vi "SUPERMARKET PROJECT SAVE DATA TO EXCEL.vi"() -> ()   [LabVIEW 2021]
uses:
  <vilib>/Utility/file.llb/Write Delimited Spreadsheet (string).vi
panel:
  in  "?":enum32{"Page 1", "Page 2"}(tab)
  in  "OK Button":bool
  in  "Username":string
  in  "Password":string
  in  "file path (dialog if empty) 2":path
  in  "stop":bool
  in  "Number 01":dbl
  in  "Number 02":dbl
  out "Answer":dbl
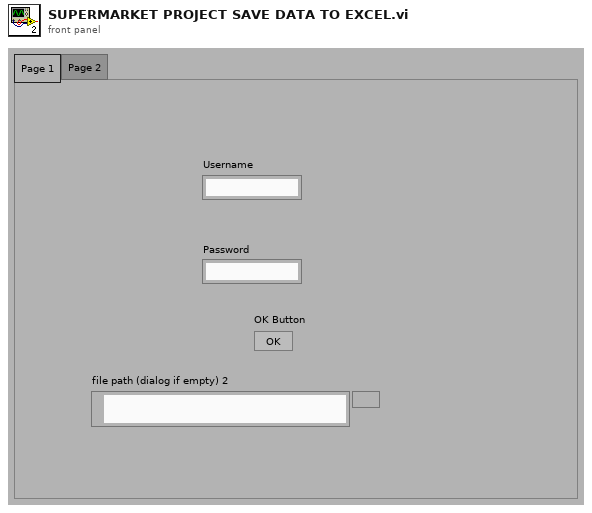
[diagram p1: front panel]
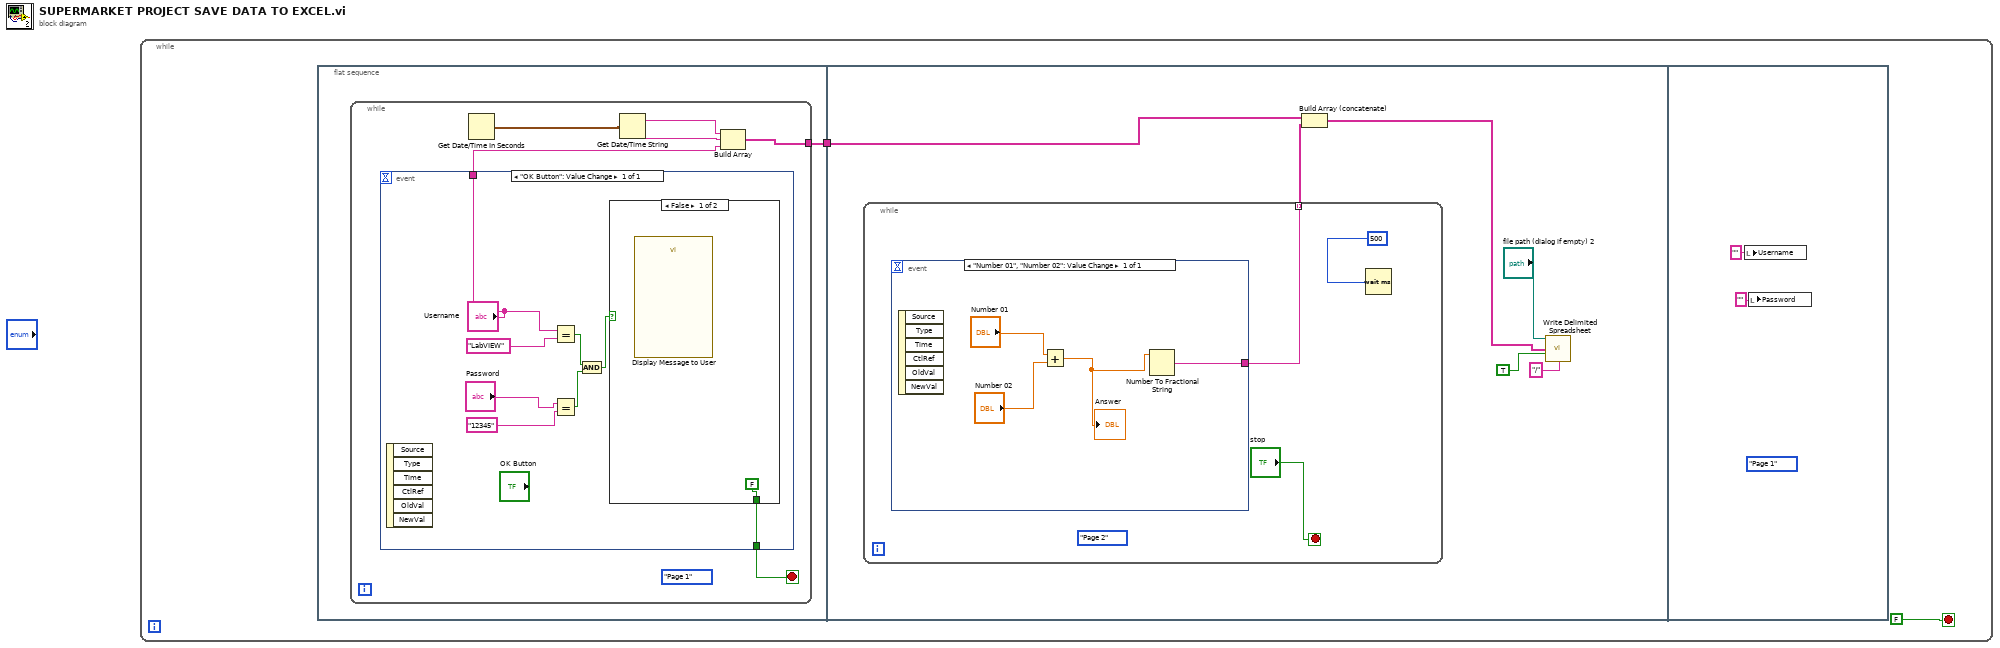
[diagram p0: block diagram]
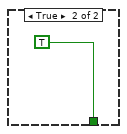
[diagram p2: hidden frame]
diagram:
  n1 = while {
    stop <- FALSE stop-if-true
    n2 = flat-sequence {
      tunnel: [w3] -> w1
      tunnel: w1 -> [w25]
      frame #0 {
        n3 = while {
          tunnel: [w7] -> w3
          stop <- w5 stop-if-true
          (unwired) enum32{"Page 1", "Page 2"}."Page 1"
          n4 = event shown="[0] \"OK Button\": Value Change" {
            selector: _ -> [_]
            dyn-events: _ -> [_]
            timeout: _ -> [_]
            tunnel: ["Username"] -> w4
            tunnel: [w10] -> w5
            event "OK Button": Value Change {
              n5 = event-data() -> ()  [unwired: 1 in, 6 out]
              n6 = Equal?(x="Username", y="LabVIEW") -> (x = y?=w14:bool)
              n7 = Equal?(x="Password", y="12345") -> (x = y?=w13:bool)
              n8 = And(x=w14, y=w13) -> (x .and. y?=w15:bool)
              n9 = case shown="False" w15 {
                tunnel: [FALSE TRUE] -> w10
                frame False {
                  n10 = call "Display Message to User"() -> ()  [unwired: 10 in, 2 out]
                }
                frame True {
                }
              }
            }
          }
          n11 = Get Date/Time In Seconds() -> (seconds since 1Jan1904=w9:timestamp)
          n12 = Get Date/Time String(seconds (now)=w9) -> (date string=w8:string, time string=w6:string)  [unwired: 2 in]
          n13 = Build Array(w8, w6, w4) -> (w7:string[])
        }
      }
      frame #1 {
        n14 = while {
          tunnel: [w27] -> w24 mode=indexing
          stop <- "stop" stop-if-true
          (unwired) enum32{"Page 1", "Page 2"}."Page 2"
          n15 = event shown="[0] \"Number 01\", \"Number 02\": Value Change" {
            selector: _ -> [_]
            dyn-events: _ -> [_]
            timeout: _ -> [_]
            tunnel: [w29] -> w27
            event "Number 01", "Number 02": Value Change {
              n16 = event-data() -> ()  [unwired: 1 in, 6 out]
              n17 = Add(x="Number 01", y="Number 02") -> (x+y=w30:dbl)
              "Answer" <- w30
              n18 = Number To Fractional String(number=w30) -> (F-format string=w29:string)  [unwired: 3 in]
            }
          }
          n19 = Wait (ms)(milliseconds to wait=u32 500) -> ()  [unwired: 1 out]
        }
        n20 = Build Array (concatenate)(w25, w24) -> (w21:string[])
        n21 = call-poly <vilib>:"Write Delimited Spreadsheet.vi"("file path (dialog if empty)"="file path (dialog if empty) 2", "1D data"=w21, "append to file? (new file:F)"=TRUE, "delimiter (\\t)"="/" ("delimiter (\\t)")) -> ()  [unwired: 10 in, 2 out]
      }
      frame #2 {
        (unwired) enum32{"Page 1", "Page 2"}."Page 1"
        n22 = local write "Username"("" ("Username")) -> ()
        n23 = local write "Password"("" ("Password")) -> ()
      }
    }
  }
